vi "Alias or Channel Lookup.vi"(8 "error in (no error)":errorcluster, 10 "Item":string, 11 "WorkspaceManager in":T1) -> (0 "error out":errorcluster, 1 "Channel":string, 2 "Alias":string, 3 "WorkspaceManager out":T1)   [LabVIEW 2011]
uses:
  <vilib>/NI Veristand/Execution/Workspace/WorkspaceAPI.ctl
  NationalInstruments.VeriStand.ClientAPI
  <vilib>/NI Veristand/Execution/Workspace/NI_VS Workspace ExecutionAPI.lvlib
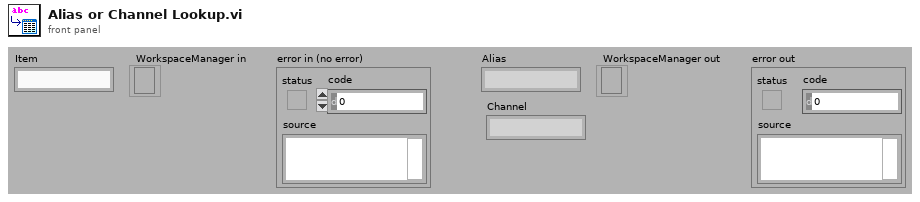
[diagram p1: front panel]
types:
  T1 = typedef "NI_VS Workspace ExecutionAPI.lvlib/WorkspaceAPI.ctl" = refnum<k24>
  T2 = typedef "NI_VS Workspace ExecutionAPI.lvlib/NodeInfo.ctl" = cluster{"Name":string, "FullPath":string, "Type":string, "IsChannel":bool, "Channel":cluster{"Unit":string, "Readable":bool, "Writable":bool, "Faultable":bool, "Scalable":bool, "RowDim":u32, "ColumnDim":u32}}
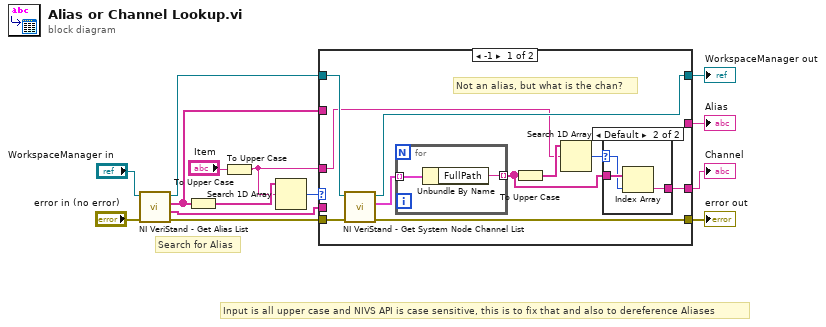
[diagram p0: block diagram]
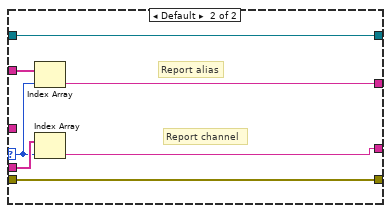
[diagram p3: hidden frame]
diagram:
  # "Input is all upper case and NIVS API is case sensitive, this is to fix that and also to dereference Aliases"
  # "Search for Alias"
  n1 = call <vilib>:"NI VeriStand - Get Alias List.vi"("error in (no error)"="error in (no error)", "WorkspaceManager in"="WorkspaceManager in") -> ("error out"=w8:errorcluster, "Channels"=w3:string[], "Aliases"=w10:string[], "WorkspaceManager out"=w7:T1)  [unwired: 6 in]
  n2 = To Upper Case(1:w10) -> (0:w14:string[])
  n3 = To Upper Case(1:"Item") -> (0:w1:string)
  n4 = Search 1D Array(1D array=w14, element=w1) -> (index of element=w13:i32)  [unwired: 1 in]
  n5 = case shown="-1" w13 {
    selector: w13 -> [_ w33]
    tunnel: w10 -> [_ w36]
    tunnel: w1 -> [w16 _]
    tunnel: [_ w35] -> w9
    tunnel: w8 -> [w21 w31]
    tunnel: w7 -> [w20 w30]
    tunnel: [w19 w30] -> w6
    tunnel: [w18 w31] -> w5
    tunnel: [w17 w32] -> w4
    tunnel: w3 -> [_ w34]
    frame -1 {
      # "Not an alias, but what is the chan?"
      n6 = call <vilib>:"NI VeriStand - Get System Node Channel List.vi"("error in (no error)"=w21, "WorkspaceManager in"=w20) -> ("error out"=w18:errorcluster, "Channels"=w22:T2[], "WorkspaceManager out"=w19:T1)  [unwired: 7 in]
      n7 = for {
        tunnel: w22 -> [w29] mode=indexing
        tunnel: [w28] -> w15 mode=indexing
        n8 = Unbundle By Name(w29) -> ("FullPath"=w28:string)
      }
      n9 = To Upper Case(1:w15) -> (0:w24:string[])
      n10 = Search 1D Array(1D array=w24, element=w16) -> (index of element=w23:i32)  [unwired: 1 in]
      n11 = case shown="Default" w23 {
        selector: w23 -> [_ w26]
        tunnel: w15 -> [_ w27]
        tunnel: [_ w25] -> w17
        frame -1 {
        }
        frame Default {
          n12 = Index Array(array=w27, index=w26) -> (element=w25:string)
        }
      }
    }
    frame Default {
      # "Report channel"
      # "Report alias"
      n13 = Index Array(array=w36, index=w33) -> (element=w35:string)
      n14 = Index Array(array=w34, index=w33) -> (element=w32:string)
    }
  }
  "Alias" <- w9
  "error out" <- w5
  "WorkspaceManager out" <- w6
  "Channel" <- w4
